vi "Collapse All.vi"(11 "UI Data in":refnum<class "Settings UI.lvclass">) -> (3 "UI Data out":refnum<class "Settings UI.lvclass">)   [LabVIEW 2020, in "Output Sequencer.lvlib" / "Settings UI.lvclass"]
uses:
  Settings UI.lvclass
  Types/Tree Index Enum.ctl
  Settings UI.lvclass/Settings UI.ctl
  Globals/Global Tree Data.vi
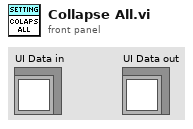
[diagram p1: front panel]
types:
  T1 = typedef "Output Sequencer.lvlib/Settings UI.lvclass/Tree Index Enum.ctl" = enum16{"General Settings", "Num Steps", "Num Analog", "Num Digital", "Show Confirmation", "Interp Priority", "Adv Timing", "Enable Conditions", "Seq Execution", "Reset Test Start", "Only When Test", "Delay After Test", "Start condition", "Re-triggering", "Stop condition", "Stop After Cycles", "Stop Values", "Default Values", "Default Analog", "Default Digital", "Steps", "Step #", "Description", "Precondition", "Duration", "Mode", "Delay Between Vals", "Analog Values", "Digital Values", "Postcondition", "On True", "On False"}
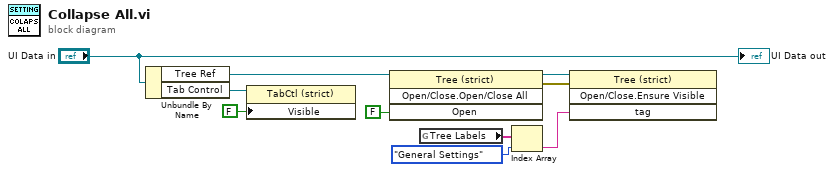
[diagram p0: block diagram]
diagram:
  n1 = Unbundle By Name("UI Data in") -> ("Tree Ref"=w9:refnum<vi>, "Tab Control"=w3:refnum<vi>)
  n2 = property class="TabCtl (strict)"(reference=w3, "Visible"=FALSE) -> ()  [unwired: 1 in, 2 out]
  n3 = invoke on="Invoke Node" class="Tree (strict)" method="Open/Close.Open/Close All"(reference=w9, "Open"=FALSE ("Open?")) -> (reference out=w7:refnum<vi>, error out=w6:errorcluster)  [unwired: 2 in, 2 out]
  n4 = global read "Global Tree Data.vi" "Tree Labels"() -> (w5:string[])
  n5 = Index Array(array=w5, index=Tree_Index_Enum."General Settings" ("Tree Index Enum")) -> (element=w4:string)
  n6 = invoke on="Invoke Node" class="Tree (strict)" method="Open/Close.Ensure Visible"(reference=w7, error in=w6, "tag"=w4) -> ()  [unwired: 1 in, 4 out]
  "UI Data out" <- "UI Data in"
